vi "Aug_CFG_to_String.vi"(11 "Config":cluster{"Flip?":bool, "Rotation":T1}) -> (3 "Aug_Name":string="FR020")   [LabVIEW 2020]
uses:
  Controls/Aug_Rotation.ctl
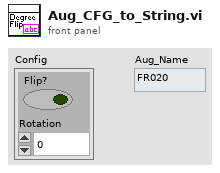
[diagram p1: front panel]
types:
  T1 = typedef "Aug_Rotation.ctl" = enum16{"0", "90", "180", "270"}
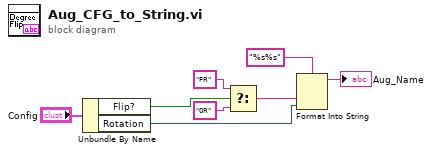
[diagram p0: block diagram]
diagram:
  n1 = Unbundle By Name("Config") -> ("Flip?"=w3:bool, "Rotation"=w2:T1)
  n2 = Select(t="FR", s=w3, f="0R") -> (s? t:f=w6:string)
  n3 = Format Into String(format string="%s%s", w6, w2) -> (resulting string=→"Aug_Name":string)  [unwired: 2 in, 1 out]
